vi "Command Loop - Apply Config.vi"(8 "error in":errorcluster, 10 "Data":u8[](array[numeric]), 11 "Queue Refs in":variant) -> (0 "error out":errorcluster, 2 "Response":string, 3 "Queue Refs out":variant)   [LabVIEW 2026, in "Runtime Configuration Support Example Engine.lvlib"]
uses:
  Runtime Configuration Support Example Engine.lvlib
  Shared/Compiled.Settings.ctl
  <vilib>/NI VeriStand/Custom Device API/Custom Device Item Ref.ctl
  <vilib>/NI VeriStand/Custom Device API/Custom Device API.lvlib
  Shared/Runtime Configuration Support Example Shared.lvlib
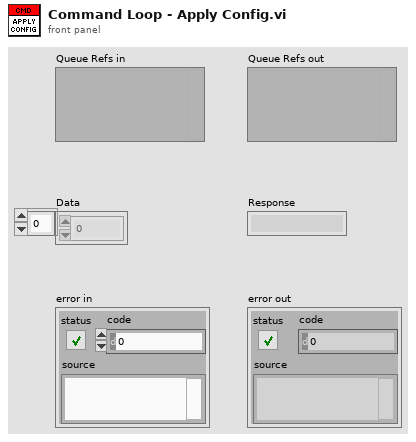
[diagram p1: front panel]
types:
  T1 = cluster{"Compiled Info":refnum<queue>, "Set HW Val Ref":refnum<queue>, "Get HW Val Ref":refnum<queue>}
  T2 = cluster{"Dynamic Config Status":bool, "Inports":i32[], "Outports":i32[], "Error":errorcluster}
  T3 = typedef "Runtime Configuration Support Example Shared.lvlib/Compiled.Settings.ctl" = cluster{"Name":string, "Inport SignalIDs":i32[], "Outport SignalIDs":i32[], "Inport Channel refs":T4[], "Outport Channel refs":T4[], "Inport Values":dbl[], "Outport Values":dbl[], "Device Error":errorcluster, "Dynamic Config Status":bool, "Response Ref":refnum<queue>}
  T4 = typedef "Custom Device API.lvlib/Custom Device Item Ref.ctl" = u64
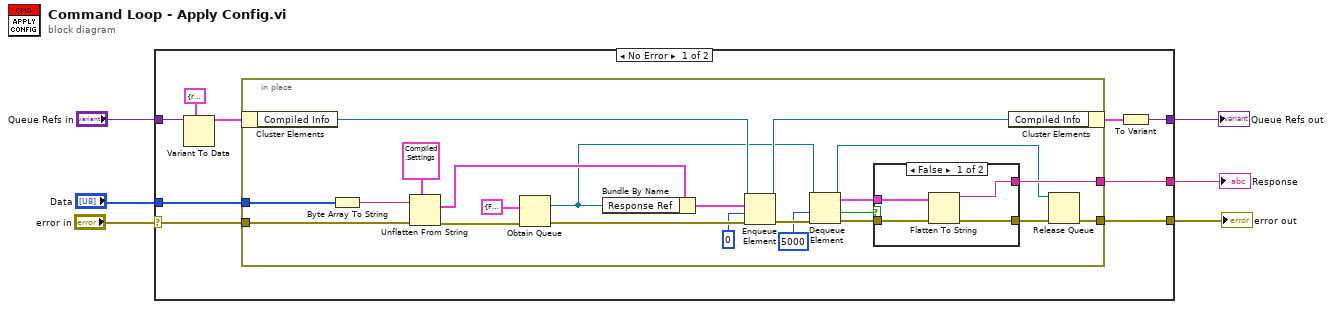
[diagram p0: block diagram]
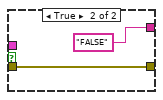
[diagram p2: hidden frame]
diagram:
  n1 = case shown="No Error" "error in" {
    selector: "error in" -> [w14 w45]
    tunnel: [w15 w45] -> w6
    tunnel: "Data" -> [w13 _]
    tunnel: [w12 _] -> w3
    tunnel: "Queue Refs in" -> [w10 w44]
    tunnel: [w7 w44] -> w2
    frame No Error {
      n2 = Variant To Data(type=T1 {"Compiled Info"=refnum, "Set HW Val Ref"=refnum, "Get HW Val Ref"=refnum} ("Queue Refs"), Variant=w10) -> (data=w11:T1)  [unwired: 1 in, 1 out]
      n3 = in-place {
        in-place-border: [w31] -> w15
        in-place-border: w14 -> [w34]
        in-place-border: w13 -> [w26]
        in-place-border: [w23] -> w12
        n4 = in-place-cluster #1(w11) -> ("Compiled Info"=w21:refnum<queue>)
        n5 = Byte Array To String(unsigned byte array=w26) -> (string=w27:string)
        n6 = Unflatten From String(type=T3 {"Name"="", "Inport SignalIDs"=[], "Outport SignalIDs"=[], "Inport Channel refs"=[], "Outport Channel refs"=[], "Inport Values"=[], "Outport Values"=[], "Device Error"={"status"=FALSE, "code"=0, "source"=""}, "Dynamic Config Status"=FALSE, "Response Ref"=refnum} ("Compiled.Settings"), binary string=w27, error in (no error)=w34) -> (value=w29:T3, error out=w37:errorcluster)  [unwired: 2 in, 1 out]
        n7 = Obtain Queue(element data type=T2 {"Dynamic Config Status"=FALSE, "Inports"=[], "Outports"=[], "Error"={"status"=FALSE, "code"=0, "source"=""}}, error in (no error)=w37) -> (queue out=w18:refnum<queue>, error out=w36:errorcluster)  [unwired: 3 in, 1 out]
        n8 = Bundle By Name(cluster=w29, "Response Ref"=w18) -> (w30:T3)
        n9 = Enqueue Element(queue=w21, element=w30, timeout in ms (-1)=0, error in (no error)=w36) -> (queue out=w20:refnum<queue>, error out=w33:errorcluster)  [unwired: 1 out]
        n10 = Dequeue Element(queue=w18, timeout in ms (-1)=5000, error in (no error)=w33) -> (queue out=w17:refnum<queue>, element=w25:T2, timed out?=w24:bool, error out=w35:errorcluster)
        n11 = case shown="False" w24 {
          tunnel: w25 -> [w38 _]
          tunnel: [w39 "FALSE"] -> w23
          tunnel: w35 -> [w41 w43]
          tunnel: [w40 w43] -> w32
          frame False {
            n12 = Flatten To String(anything=w38, error in (no error)=w41) -> (data string=w39:string, error out=w40:errorcluster)  [unwired: 2 in, 1 out]
          }
          frame True {
          }
        }
        n13 = in-place-cluster #1("Compiled Info"=w20) -> (w8:T1)
        n14 = Release Queue(queue=w17, error in (no error)=w32) -> (error out=w31:errorcluster)  [unwired: 1 in, 2 out]
      }
      n15 = To Variant(anything=w8) -> (Variant=w7:variant)
    }
    frame Error {
    }
  }
  "error out" <- w6
  "Response" <- w3
  "Queue Refs out" <- w2
